vi "Read Measurement (Statistics).vi"(8 "error in (no error)":errorcluster, 10 "Timeout (10000 ms)":u32=10000, 11 "VISA resource name":refnum<visa-resource-name>) -> (0 "error out":errorcluster, 1 "Standard Deviation":dbl, 2 "Mean":dbl format="%#_12g", 3 "VISA resource name out":refnum<visa-resource-name>, 4 "Maximum":dbl format="%#_12g", 5 "Minimum":dbl format="%#_12g")   [LabVIEW 2024, in "Agilent 532XX Series.lvlib"]
doc: "Performs a single, new measurement and outputs measurement statistics."
uses:
  Agilent 532XX Series.lvlib
  Low Level/Fetch Measurement (Statistics).vi
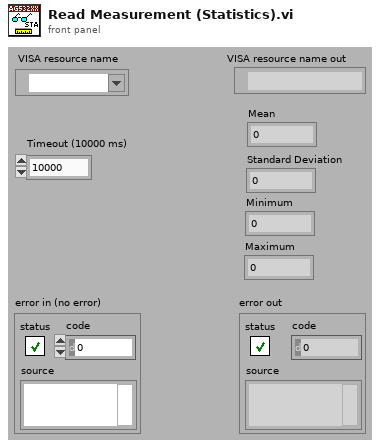
[diagram p1: front panel]
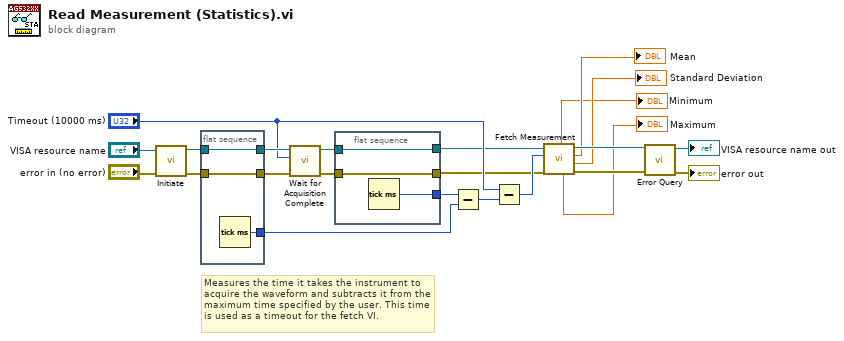
[diagram p0: block diagram]
diagram:
  # "Measures the time it takes the instrument to acquire the waveform and subtracts it from the maximum time specified by the user. This time is used as a timeout for the fetch VI."
  n1 = call "Initiate.vi"("error in (no error)"="error in (no error)", "VISA resource name"="VISA resource name") -> ("error out"=w17:errorcluster, "VISA resource name out"=w18:refnum<visa-resource-name>)  [unwired: 8 out]
  n2 = flat-sequence {
    tunnel: [w26] -> w14
    tunnel: w18 -> [w26]
    tunnel: [w25] -> w15
    tunnel: w17 -> [w25]
    tunnel: [w24] -> w16
    frame #0 {
      n3 = Tick Count (ms)() -> (millisecond timer value=w24:u32)
    }
  }
  n4 = call "Wait for Acquisition Complete.vi"("error in (no error)"=w15, "Maximum Time (10000 ms)"="Timeout (10000 ms)", "VISA resource name"=w14) -> ("error out"=w11:errorcluster, "VISA resource name out"=w12:refnum<visa-resource-name>)  [unwired: 1 in, 6 out]
  n5 = flat-sequence {
    tunnel: [w29] -> w7
    tunnel: w12 -> [w29]
    tunnel: [w28] -> w8
    tunnel: w11 -> [w28]
    tunnel: [w27] -> w10
    frame #0 {
      n6 = Tick Count (ms)() -> (millisecond timer value=w27:u32)
    }
  }
  n7 = Subtract(x=w10, y=w16) -> (x-y=w19:u32)
  n8 = Subtract(x="Timeout (10000 ms)", y=w19) -> (x-y=w9:u32)
  n9 = call-poly "Fetch Measurement.vi"("error in (no error)"=w8, "Timeout (10000 ms)"=w9, "VISA resource name"=w7) -> ("error out"=w5:errorcluster, "Standard Deviation"=→"Standard Deviation":dbl, "Mean"=→"Mean":dbl, "VISA resource name out"=w6:refnum<visa-resource-name>, "Maximum"=→"Maximum":dbl, "Minimum"=→"Minimum":dbl)  [unwired: 3 out]
  n10 = call "Error Query.vi"("error in (no error)"=w5, "VISA resource name"=w6) -> ("error out"=→"error out":errorcluster, "VISA resource name out"=→"VISA resource name out":refnum<visa-resource-name>)  [unwired: 8 out]
